vi "Convert to DataGrid String.vi"(10 "Display Style":T1, 11 "Popup String in":string) -> (3 "DataGrid String out":string)   [LabVIEW 2018, in "String Data Type.lvclass"]
uses:
  String Data Type.lvclass
  Display Style Enum.ctl
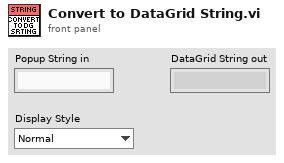
[diagram p1: front panel]
types:
  T1 = typedef "String Data Type.lvclass/Display Style Enum.ctl" = enum16{"Normal", "'\\' Codes", "Hex"}
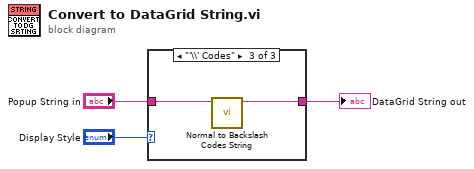
[diagram p0: block diagram]
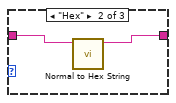
[diagram p3: hidden frame]
diagram:
  n1 = case shown="\"'\\\\' Codes\"" "Display Style" {
    tunnel: "Popup String in" -> [w4 w6 w8]
    tunnel: [w4 w5 w7] -> w3
    frame "Normal" {
    }
    frame "Hex" {
      n2 = call "Normal to Hex String.vi"("Normal String in"=w6) -> ("Hex String out"=w5:string)  [unwired: 10 in]
    }
    frame "'\\' Codes" {
      n3 = call "Normal to Backslash Codes String.vi"("Normal String in"=w8) -> ("Backslash String out"=w7:string)  [unwired: 10 in]
    }
  }
  "DataGrid String out" <- w3
